vi "Z Aux Direct Cancel Axis List.vi"(7 "imode":i32, 8 "error in (no error)":errorcluster caption="错误输入（无错误）", 9 "piAxislist":i32, 10 "imaxaxises":i32, 11 "handle":u32) -> (0 "error out":errorcluster caption="错误输出", 1 "piAxislist out":i32, 2 "function return":i32, 3 "handle out":u32)   [LabVIEW 2015, in "zauxdll.lvlib"]
doc: "int32 __stdcall ZAux_Direct_CancelAxisList(ZMC_HANDLE handle, int imaxaxises, int *piAxislist, int imode);"
uses:
  zauxdll.lvlib
  zauxdll.dll
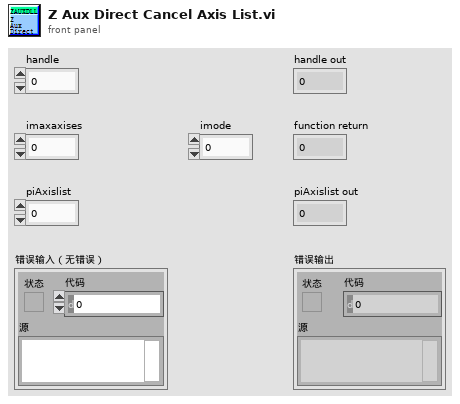
[diagram p1: front panel]
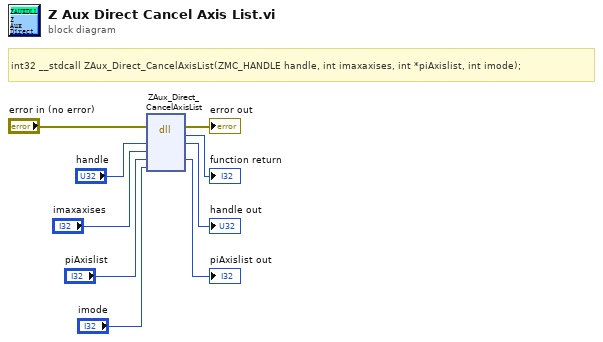
[diagram p0: block diagram]
diagram:
  # "int32 __stdcall ZAux_Direct_CancelAxisList(ZMC_HANDLE handle, int imaxaxises, int *piAxislist, int imode);"
  n1 = dll-call lib="C:/Users/VIC/Desktop/GOGORO_Oringnal - Panasonic/system/LLB/zmotion/zaux/zauxdll.*" fn="ZAux_Direct_CancelAxisList"(error in="error in (no error)", "handle"="handle", "imaxaxises"="imaxaxises", "piAxislist"="piAxislist", "imode"="imode") -> (error out=→"error out":errorcluster, →"function return":i32, "handle"=→"handle out":u32, "piAxislist"=→"piAxislist out":i32)  [unwired: 4 in, 1 out]
